vi "check engine status.vi"(8 "error in (no error)":errorcluster, 11 "engine status":T4(array[cluster])) -> (0 "error out":errorcluster, 3 "JSON string":string)   [LabVIEW 2014]
uses:
  <vilib>/NI/Module Execution Interface/Engine Runtime/Execution States.ctl
  <vilib>/NI/Module Execution Interface/Engine Runtime/Fault.ctl
  <vilib>/NI/Tag Bus Module Framework/runtime/error classification.ctl
  <vilib>/NI/Tag Bus Module Framework/runtime/TBM module execution interface.lvclass
  <vilib>/NI/Module Execution Interface/Engine Runtime/Engine Runtime Interface.lvclass
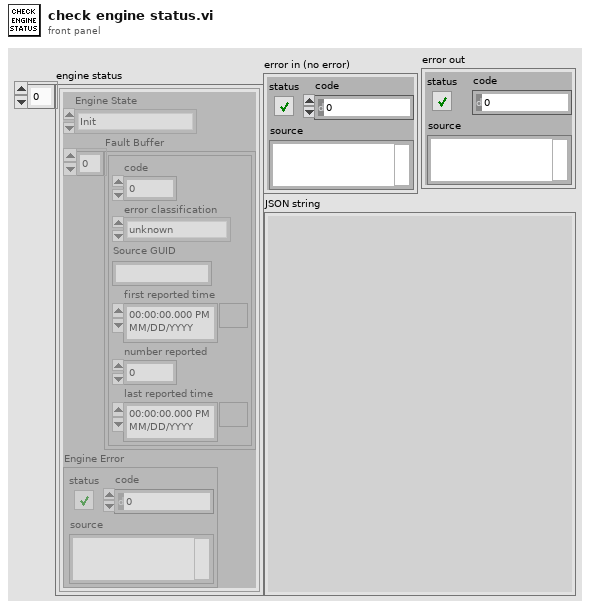
[diagram p1: front panel]
types:
  T1 = typedef "Engine Runtime Interface.lvclass/Execution States.ctl" = enum16{"Init", "Pre-Operational", "Safe-Operational", "Operational", "Stopped"}
  T2 = typedef "Engine Runtime Interface.lvclass/Fault.ctl" = cluster{"code":i32, "error classification":T3, "Source GUID":string, "first reported time":timestamp, "number reported":u32, "last reported time":timestamp}
  T3 = typedef "TBM module execution interface.lvclass/error classification.ctl" = enum16{"unknown", "none", "trivial", "recoverable", "critical"}
  T4 = cluster{"Engine State":T1, "Fault Buffer":T2[], "Engine Error":errorcluster}[]
  T5 = cluster{"fault buffer":cluster{"code":i32, "Source GUID":string, "number reported":u32, "error classification":string, "engine state":string}[], "error":errorcluster, "engine state":string}
  T6 = cluster{"code":i32, "Source GUID":string, "number reported":u32, "error classification":string, "engine state":string}
  T7 = cluster{"status":bool, "code":bool, "source":bool}
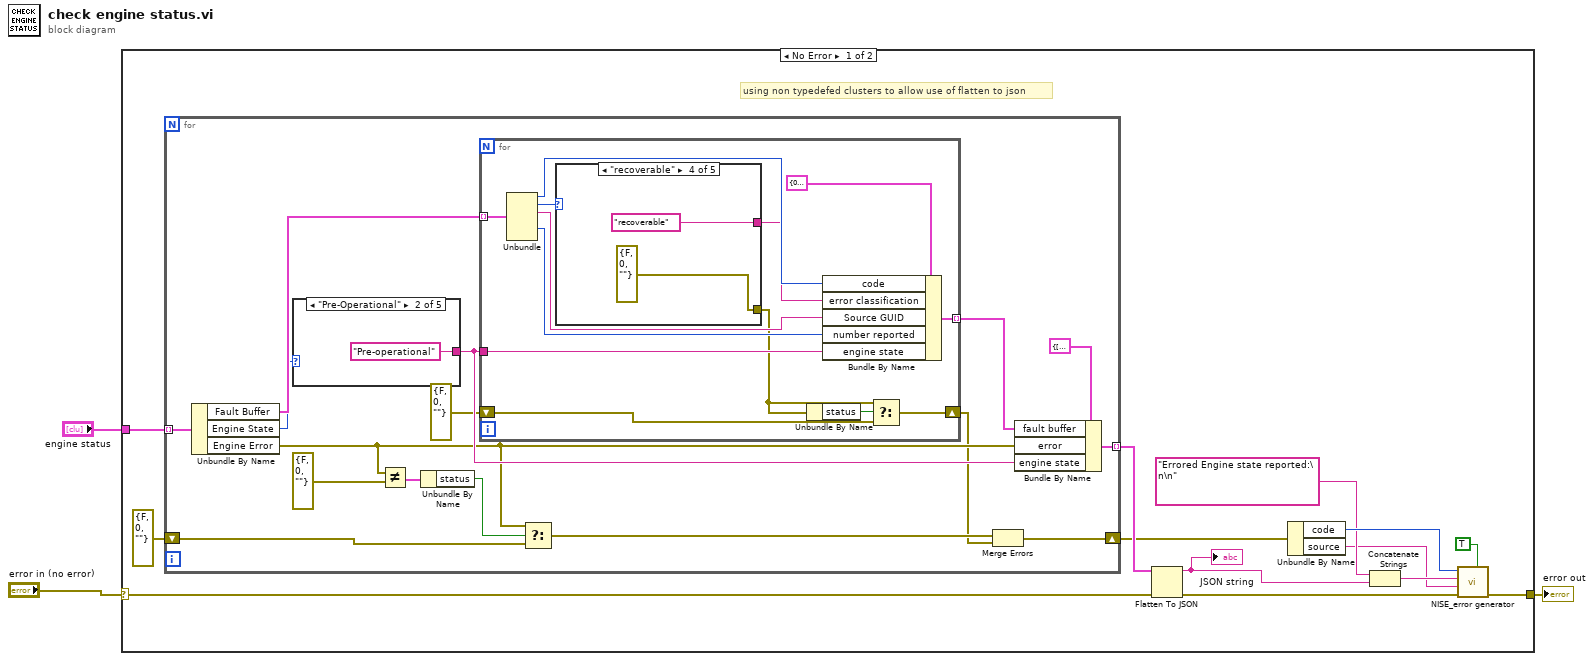
[diagram p0: block diagram]
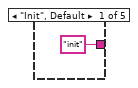
[diagram p2: hidden frame]
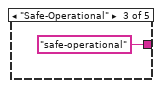
[diagram p3: hidden frame]
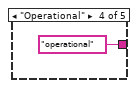
[diagram p4: hidden frame]
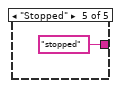
[diagram p5: hidden frame]
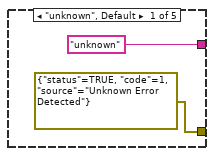
[diagram p6: hidden frame]
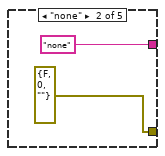
[diagram p7: hidden frame]
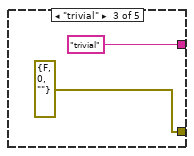
[diagram p8: hidden frame]
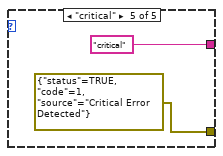
[diagram p9: hidden frame]
diagram:
  n1 = case shown="No Error" "error in (no error)" {
    selector: "error in (no error)" -> [w14 w61]
    tunnel: "engine status" -> [w16 _]
    tunnel: [w12 w61] -> w1
    frame No Error {
      # "using non typedefed clusters to allow use of flatten to json"
      n2 = for {
        tunnel: w16 -> [w32] mode=indexing
        tunnel: [w26] -> w15 mode=indexing
        shift-right: [w18] -> w9
        shift-left: errorcluster {"status"=FALSE, "code"=0, "source"=""} ("y") -> [w23]
        n3 = Unbundle By Name(w32) -> ("Fault Buffer"=w31:T2[], "Engine State"=w30:T1, "Engine Error"=w21:errorcluster)
        n4 = case shown="\"Pre-Operational\"" w30 {
          tunnel: ["init" "Pre-operational" "safe-operational" "operational" "stopped"] -> w27
          frame "Init", Default {
          }
          frame "Pre-Operational" {
          }
          frame "Safe-Operational" {
          }
          frame "Operational" {
          }
          frame "Stopped" {
          }
        }
        n5 = Not Equal?(x=w21, y=errorcluster {"status"=FALSE, "code"=0, "source"=""}) -> (x != y?=w25:T7)
        n6 = Unbundle By Name(w25) -> ("status"=w24:bool)
        n7 = for {
          tunnel: w31 -> [w50] mode=indexing
          tunnel: w27 -> [w43]
          tunnel: [w42] -> w28 mode=indexing
          shift-right: [w41] -> w17
          shift-left: errorcluster {"status"=FALSE, "code"=0, "source"=""} ("y") -> [w40]
          n8 = Unbundle(w50) -> ("code"=w48:i32, "error classification"=w45:T3, "Source GUID"=w47:string, "number reported"=w46:u32)  [unwired: 2 out]
          n9 = case shown="\"recoverable\"" w45 {
            tunnel: ["unknown" "none" "trivial" "recoverable" "critical"] -> w44
            tunnel: [errorcluster {"status"=TRUE, "code"=1, "source"="Unknown Error Detected"} ("y") errorcluster {"status"=FALSE, "code"=0, "source"=""} ("y") errorcluster {"status"=FALSE, "code"=0, "source"=""} ("y") errorcluster {"status"=FALSE, "code"=0, "source"=""} ("y") errorcluster {"status"=TRUE, "code"=1, "source"="Critical Error Detected"} ("y")] -> w38
            frame "unknown", Default {
            }
            frame "none" {
            }
            frame "trivial" {
            }
            frame "recoverable" {
            }
            frame "critical" {
            }
          }
          n10 = Unbundle By Name(w38) -> ("status"=w39:bool)
          n11 = Bundle By Name(cluster=T6 {"code"=0, "Source GUID"="", "number reported"=0, "error classification"="", "engine state"=""}, "code"=w48, "error classification"=w44, "Source GUID"=w47, "number reported"=w46, "engine state"=w43) -> (w42:T6)
          n12 = Select(t=w38, s=w39, f=w40) -> (s? t:f=w41:errorcluster)
        }
        n13 = Select(t=w21, s=w24, f=w23) -> (s? t:f=w19:errorcluster)
        n14 = Merge Errors(w19, w17) -> (w18:errorcluster)
        n15 = Bundle By Name(cluster=T5 {"fault buffer"=[], "error"={"status"=FALSE, "code"=0, "source"=""}, "engine state"="Pre-operational"}, "fault buffer"=w28, "error"=w21, "engine state"=w27) -> (w26:T5)
      }
      n16 = Flatten To JSON(anything=w15, error in (no error)=w14) -> (JSON string=w5:string, 11:w11:errorcluster)  [unwired: 1 in]
      "JSON string" <- w5
      n17 = Unbundle By Name(w9) -> ("code"=w8:i32, "source"=w4:string)
      n18 = Concatenate Strings("Errored Engine state reported:\n\n" ("append error message"), w5) -> (w7:string)
      n19 = call <vilib>:"NISE_error generator.vi"("concatenate (F)"=TRUE, "error in"=w11, "source"=w4, "append error message"=w7, "error code (0)"=w8) -> ("error out"=w12:errorcluster)  [unwired: 4 in]
    }
    frame Error {
    }
  }
  "error out" <- w1
